vi "continuous_volumetric_scan.vi"() -> ()   [LabVIEW 2017]
uses:
  <vilib>/DAQmx/write.llb/DAQmx Write (Analog DBL 1Chan 1Samp).vi
  <vilib>/DAQmx/write.llb/DAQmx Write (Analog 1D DBL NChan 1Samp).vi
  <vilib>/DAQmx/write.llb/DAQmx Write (Analog 2D DBL NChan NSamp).vi
  <vilib>/DAQmx/create/channels.llb/DAQmx Create Channel (AO-Voltage-Basic).vi
  <vilib>/DAQmx/miscellaneous.llb/DAQmx Fill In Error Info.vi
  <vilib>/Utility/file.llb/Read Delimited Spreadsheet (DBL).vi
  <vilib>/measure/mascope.llb/Transition Measurements 1 chan.vi
  <vilib>/DAQmx/configure/timing.llb/DAQmx Timing (Sample Clock).vi
  <vilib>/DAQmx/configure/trigger.llb/DAQmx Start Trigger (Digital Edge).vi
  <vilib>/measure/NI_MAPro.lvlib
panel:
  out "Sampling rate":i32
  out "ETL3":waveform(dbl)(graph)
  out "mirror y":waveform(dbl)(graph)
  out "mirror x":waveform(dbl)(graph)
  out "561":waveform(dbl)(graph)
  out "488":waveform(dbl)(graph)
  out "camera":waveform(dbl)(graph)
  out "mirx transition duration":dbl
  out "transition duration":dbl
  out "etl3 timing array":dbl[](array[numeric])
  out "mirror y timing array":dbl[](array[numeric])
  out "mirror x timing array":dbl[](array[numeric])
  out "561 timing array":dbl[](array[numeric])
  out "488 timing array":dbl[](array[numeric])
  out "camera timing array":dbl[](array[numeric])
  out "etl raw":dbl[](array[numeric])
  out "miry raw":dbl[](array[numeric])
  out "mirx raw":dbl[](array[numeric])
  out "561 Intensity":dbl
  out "488 Intensity":dbl
  out "Off Time":dbl
  out "On Time":dbl
  out "Number of slices":dbl
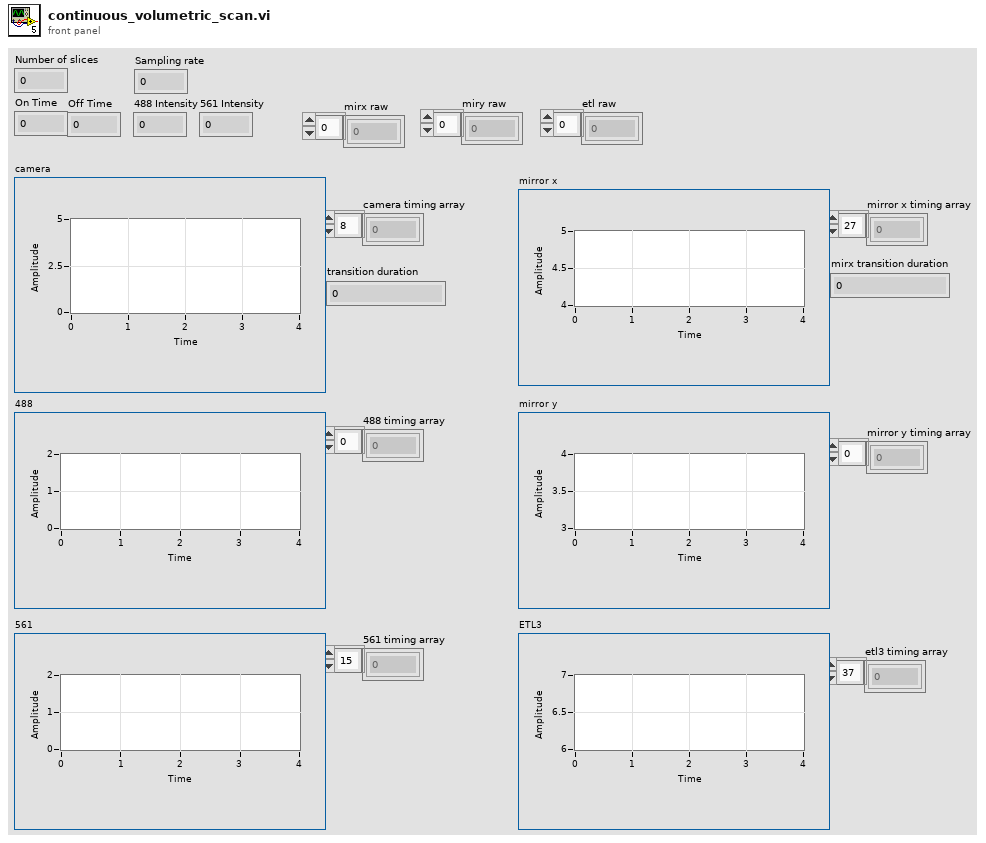
[diagram p1: front panel]
types:
  T1 = enum32{"Invalid", "Standard", "Closed", "Hidden", "Minimized", "Maximized"}
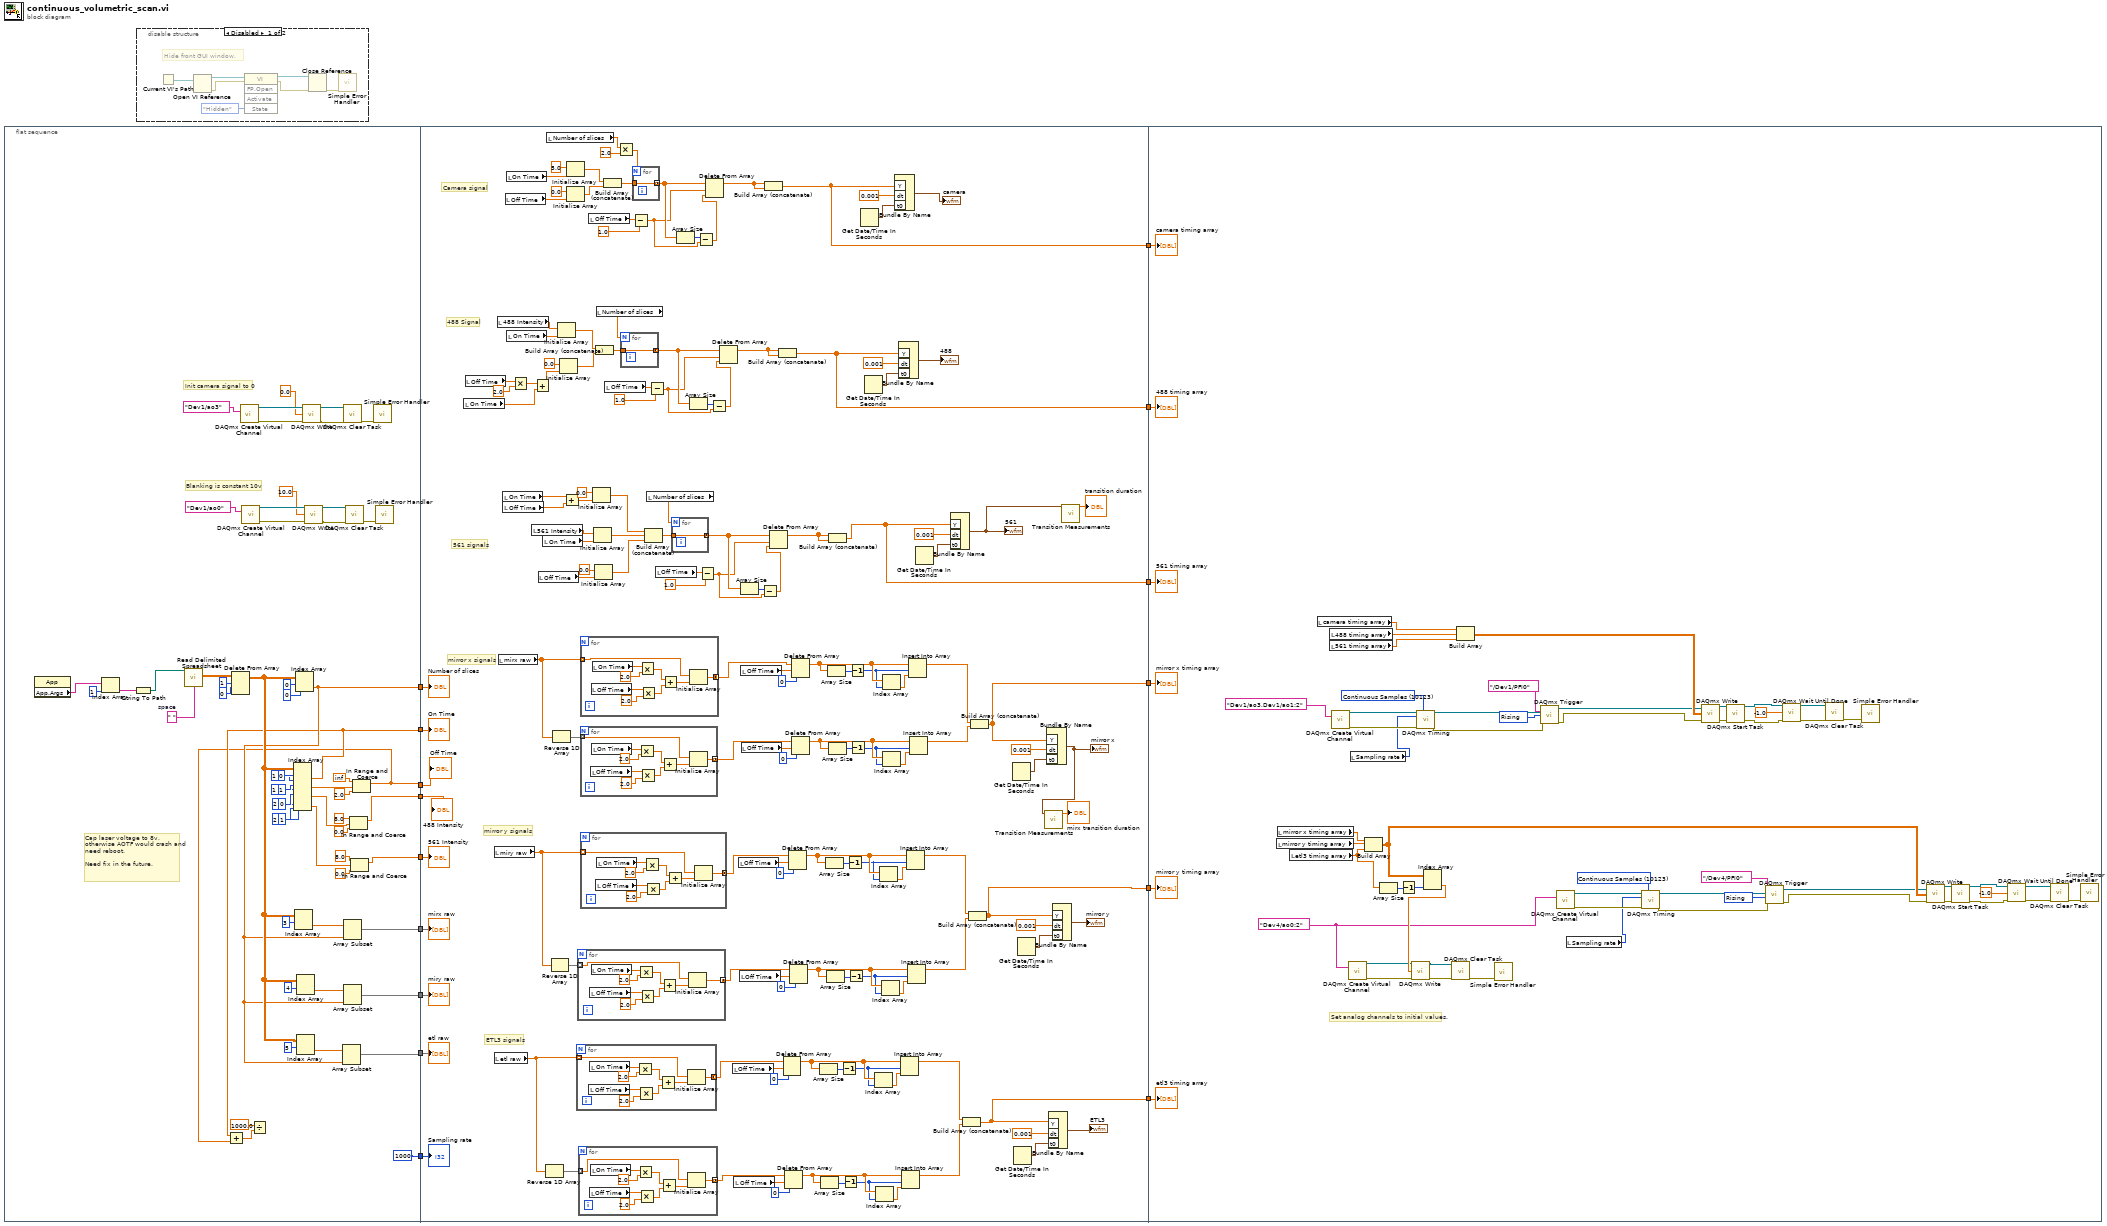
[diagram p0: block diagram]
diagram:
  n1 = flat-sequence {
    tunnel: [w50] -> w15
    tunnel: [w27] -> w14
    tunnel: [w26] -> w13
    tunnel: [w18] -> w12
    tunnel: [w16] -> w11
    tunnel: [w49] -> w10
    tunnel: [w48] -> w9
    tunnel: [w47] -> w8
    tunnel: [1000] -> w1
    tunnel: w15 -> [w97]
    tunnel: w14 -> [w96]
    tunnel: w13 -> [w95]
    tunnel: w12 -> [w94]
    tunnel: w11 -> [w93]
    tunnel: w10 -> [w92]
    tunnel: w9 -> [w91]
    tunnel: w8 -> [w90]
    tunnel: [w89] -> w7
    tunnel: [w88] -> w6
    tunnel: [w87] -> w5
    tunnel: [w86] -> w4
    tunnel: [w85] -> w3
    tunnel: [w84] -> w2
    tunnel: w1 -> [w75]
    tunnel: w7 -> [w288]
    tunnel: w6 -> [w287]
    tunnel: w5 -> [w286]
    tunnel: w4 -> [w285]
    tunnel: w3 -> [w284]
    tunnel: w2 -> [w283]
    frame #0 {
      w51 = " "  # space
      # "Cap laser voltage to 8v, otherwise AOTF would crash and need reboot. \n\nNeed fix in the future."
      # "Init camera signal to 0"
      # "Blanking is constant 10v"
      n2 = property class="App"() -> ("App.Args"=w30:string[])  [unwired: 2 in, 2 out]
      n3 = Index Array(array=w30, index=1) -> (element=w29:string)
      n4 = String To Path(string=w29) -> (path=w28:path)
      n5 = call-poly <vilib>:"Read Delimited Spreadsheet.vi"("file path (dialog if empty)"=w28, "delimiter (\\t)"=w51) -> ("all rows"=w69:dbl[][])  [unwired: 8 in, 5 out]
      n6 = Delete From Array(array=w69, length=1, index (row)=0) -> (array with subset deleted=w70:dbl[][])  [unwired: 1 in, 1 out]
      n7 = call-poly <vilib>:"DAQmx Create Virtual Channel.vi"("physical channels"=tag "Dev1/ao3") -> ("task out"=w35:refnum<k21>, "error out"=w36:errorcluster)  [unwired: 13 in]
      n8 = call-poly <vilib>:"DAQmx Create Virtual Channel.vi"("physical channels"=tag "Dev1/ao0") -> ("task out"=w43:refnum<k21>, "error out"=w44:errorcluster)  [unwired: 13 in]
      n9 = Index Array(array=w70, index (row) #1=1 ("index (row)"), index (col) #1=0 ("disabled index (col)"), index (row) #2=1 ("index (row)"), index (col) #2=1 ("disabled index (col)"), index (row) #3=2 ("index (row)"), index (col) #3=0 ("disabled index (col)"), index (row) #4=2 ("index (row)"), index (col) #4=1 ("disabled index (col)")) -> (element #1=w27:dbl, element #2=w74:dbl, element #3=w19:dbl, element #4=w17:dbl)
      n10 = Index Array(array=w70, index (row)=3) -> (element=w71:dbl[])  [unwired: 1 in]
      n11 = Index Array(array=w70, index (row)=0, index (col)=0 ("disabled index (col)")) -> (element=w50:dbl)
      n12 = Index Array(array=w70, index (row)=5) -> (element=w73:dbl[])  [unwired: 1 in]
      n13 = Index Array(array=w70, index (row)=4) -> (element=w72:dbl[])  [unwired: 1 in]
      n14 = call-poly <vilib>:"DAQmx Write.vi"("task/channels in"=w35, "data"=0.0, "error in"=w36) -> ("task out"=w37:refnum<k21>, "error out"=w38:errorcluster)  [unwired: 10 in, 1 out]
      n15 = call-poly <vilib>:"DAQmx Write.vi"("task/channels in"=w43, "data"=10.0, "error in"=w44) -> ("task out"=w45:refnum<k21>, "error out"=w46:errorcluster)  [unwired: 10 in, 1 out]
      n16 = Array Subset(array=w73, length=w50) -> (w47:dbl[])  [unwired: 1 in]
      n17 = call <vilib>:"DAQmx Clear Task.vi"("task in"=w37, "error in"=w38) -> ("error out"=w34:errorcluster)  [unwired: 13 in]
      n18 = Array Subset(array=w71, length=w50) -> (w49:dbl[])  [unwired: 1 in]
      n19 = Array Subset(array=w72, length=w50) -> (w48:dbl[])  [unwired: 1 in]
      n20 = call <vilib>:"DAQmx Clear Task.vi"("task in"=w45, "error in"=w46) -> ("error out"=w42:errorcluster)  [unwired: 13 in]
      n21 = In Range and Coerce(upper limit=8.0, x=w19, lower limit=0.0) -> (coerced(x)=w18:dbl)  [unwired: 1 out]
      n22 = In Range and Coerce(upper limit=8.0, x=w17, lower limit=0.0) -> (coerced(x)=w16:dbl)  [unwired: 1 out]
      n23 = In Range and Coerce(upper limit=inf, x=w74, lower limit=2.0) -> (coerced(x)=w26:dbl)  [unwired: 1 out]
      n24 = Add(x=w27, y=w26) -> (x+y=w24:dbl)
      n25 = Divide(x=1000.0, y=w24) -> ()  [unwired: 1 out]
      n26 = call <vilib>:"Simple Error Handler.vi"("error in (no error)"=w34) -> ()  [unwired: 4 in, 5 out]
      n27 = call <vilib>:"Simple Error Handler.vi"("error in (no error)"=w42) -> ()  [unwired: 4 in, 5 out]
    }
    frame #1 {
      # "ETL3 signals"
      # "mirror y signals"
      # "mirror x signals"
      # "561 signals"
      # "488 Signal"
      # "Camera signal"
      n28 = local read "On Time"() -> (w195:dbl)
      n29 = local read "Off Time"() -> (w198:dbl)
      n30 = local read "miry raw"() -> (w124:dbl[])
      n31 = local read "etl raw"() -> (w120:dbl[])
      n32 = local read "488 Intensity"() -> (w202:dbl)
      n33 = local read "mirx raw"() -> (w128:dbl[])
      n34 = local read "On Time"() -> (w169:dbl)
      n35 = local read "Off Time"() -> (w180:dbl)
      n36 = local read "Off Time"() -> (w217:dbl)
      n37 = local read "On Time"() -> (w218:dbl)
      n38 = local read "On Time"() -> (w201:dbl)
      n39 = Multiply(x=w198, y=2.0) -> (x*y=w196:dbl)
      n40 = local read "561 Intensity"() -> (w183:dbl)
      n41 = Add(x=w196, y=w195) -> (x+y=w194:dbl)
      n42 = local read "Off Time"() -> (w165:dbl)
      n43 = local read "On Time"() -> (w182:dbl)
      n44 = Reverse 1D Array(array=w120) -> (reversed array=w118:dbl[])
      n45 = local read "Number of slices"() -> (w210:dbl)
      n46 = Reverse 1D Array(array=w124) -> (reversed array=w122:dbl[])
      n47 = Reverse 1D Array(array=w128) -> (reversed array=w126:dbl[])
      n48 = Initialize Array(w202, w201) -> (w200:dbl[])
      n49 = Initialize Array(0.0 ("element"), w194) -> (w193:dbl[])
      n50 = Add(x=w169, y=w180) -> (x+y=w179:dbl)
      n51 = Initialize Array(5.0 ("element"), w218) -> (w215:dbl[])
      n52 = Initialize Array(0.0 ("element"), w217) -> (w214:dbl[])
      n53 = for {
        tunnel: w120 -> [w230] mode=indexing
        tunnel: [w229] -> w119 mode=concatenating
        n54 = local read "Off Time"() -> (w235:dbl)
        n55 = local read "On Time"() -> (w233:dbl)
        n56 = Multiply(x=w233, y=2.0) -> (x*y=w234:dbl)
        n57 = Multiply(x=w235, y=2.0) -> (x*y=w236:dbl)
        n58 = Add(x=w234, y=w236) -> (x+y=w237:dbl)
        n59 = Initialize Array(w230, w237) -> (w229:dbl[])
      }
      n60 = for {
        tunnel: w122 -> [w239] mode=indexing
        tunnel: [w238] -> w121 mode=concatenating
        n61 = local read "Off Time"() -> (w244:dbl)
        n62 = local read "On Time"() -> (w242:dbl)
        n63 = Multiply(x=w242, y=2.0) -> (x*y=w243:dbl)
        n64 = Multiply(x=w244, y=2.0) -> (x*y=w245:dbl)
        n65 = Add(x=w243, y=w245) -> (x+y=w246:dbl)
        n66 = Initialize Array(w239, w246) -> (w238:dbl[])
      }
      n67 = for {
        tunnel: w118 -> [w221] mode=indexing
        tunnel: [w220] -> w117 mode=concatenating
        n68 = local read "Off Time"() -> (w226:dbl)
        n69 = local read "On Time"() -> (w224:dbl)
        n70 = Multiply(x=w224, y=2.0) -> (x*y=w225:dbl)
        n71 = Multiply(x=w226, y=2.0) -> (x*y=w227:dbl)
        n72 = Add(x=w225, y=w227) -> (x+y=w228:dbl)
        n73 = Initialize Array(w221, w228) -> (w220:dbl[])
      }
      n74 = for {
        tunnel: w128 -> [w266] mode=indexing
        tunnel: [w265] -> w127 mode=concatenating
        n75 = local read "Off Time"() -> (w271:dbl)
        n76 = local read "On Time"() -> (w273:dbl)
        n77 = Multiply(x=w273, y=2.0) -> (x*y=w272:dbl)
        n78 = Multiply(x=w271, y=2.0) -> (x*y=w270:dbl)
        n79 = Add(x=w272, y=w270) -> (x+y=w269:dbl)
        n80 = Initialize Array(w266, w269) -> (w265:dbl[])
      }
      n81 = for {
        tunnel: w126 -> [w257] mode=indexing
        tunnel: [w256] -> w125 mode=concatenating
        n82 = local read "Off Time"() -> (w262:dbl)
        n83 = local read "On Time"() -> (w264:dbl)
        n84 = Multiply(x=w264, y=2.0) -> (x*y=w263:dbl)
        n85 = Multiply(x=w262, y=2.0) -> (x*y=w261:dbl)
        n86 = Add(x=w263, y=w261) -> (x+y=w260:dbl)
        n87 = Initialize Array(w257, w260) -> (w256:dbl[])
      }
      n88 = for {
        tunnel: w124 -> [w248] mode=indexing
        tunnel: [w247] -> w123 mode=concatenating
        n89 = local read "Off Time"() -> (w253:dbl)
        n90 = local read "On Time"() -> (w251:dbl)
        n91 = Multiply(x=w251, y=2.0) -> (x*y=w252:dbl)
        n92 = Multiply(x=w253, y=2.0) -> (x*y=w254:dbl)
        n93 = Add(x=w252, y=w254) -> (x+y=w255:dbl)
        n94 = Initialize Array(w248, w255) -> (w247:dbl[])
      }
      n95 = local read "Off Time"() -> (w209:dbl)
      n96 = Initialize Array(0.0 ("element"), w179) -> (w168:dbl[])
      n97 = Initialize Array(w183, w182) -> (w167:dbl[])
      n98 = Initialize Array(0.0 ("element"), w165) -> (w164:dbl[])
      n99 = Build Array (concatenate)(w200, w193) -> (w191:dbl[])
      n100 = local read "Number of slices"() -> (w192:dbl)
      n101 = Build Array (concatenate)(w215, w214) -> (w213:dbl[])
      n102 = local read "Off Time"() -> (w187:dbl)
      n103 = Multiply(x=w210, y=2.0) -> (x*y=w212:dbl)
      n104 = for {
        N: w192 -> [_]
        tunnel: w191 -> [w275]
        tunnel: [w275] -> w188 mode=concatenating
      }
      n105 = for {
        N: w212 -> [_]
        tunnel: w213 -> [w276]
        tunnel: [w276] -> w207 mode=concatenating
      }
      n106 = Subtract(x=w209, y=1.0) -> (x-y=w205:dbl)
      n107 = Build Array (concatenate)(w168, w167, w164) -> (w177:dbl[])
      n108 = local read "Number of slices"() -> (w178:dbl)
      n109 = Subtract(x=w187, y=1.0) -> (x-y=w185:dbl)
      n110 = local read "Off Time"() -> (w173:dbl)
      n111 = for {
        N: w178 -> [_]
        tunnel: w177 -> [w274]
        tunnel: [w274] -> w174 mode=concatenating
      }
      n112 = Array Size(array=w207) -> (size(s)=w206:i32)
      n113 = Array Size(array=w188) -> (size(s)=w190:i32)
      n114 = Subtract(x=w206, y=w205) -> (x-y=w204:dbl)
      n115 = Subtract(x=w173, y=1.0) -> (x-y=w171:dbl)
      n116 = Delete From Array(array=w207, length=w205, index=w204) -> (array with subset deleted=w203:dbl[])  [unwired: 1 out]
      n117 = Subtract(x=w190, y=w185) -> (x-y=w189:dbl)
      n118 = Delete From Array(array=w188, length=w185, index=w189) -> (array with subset deleted=w184:dbl[])  [unwired: 1 out]
      n119 = local read "Off Time"() -> (w139:dbl)
      n120 = local read "Off Time"() -> (w134:dbl)
      n121 = local read "Off Time"() -> (w151:dbl)
      n122 = local read "Off Time"() -> (w146:dbl)
      n123 = Array Size(array=w174) -> (size(s)=w176:i32)
      n124 = local read "Off Time"() -> (w163:dbl)
      n125 = local read "Off Time"() -> (w158:dbl)
      n126 = Subtract(x=w176, y=w171) -> (x-y=w175:dbl)
      n127 = Build Array (concatenate)(w203, w203) -> (w89:dbl[])
      n128 = Delete From Array(array=w174, length=w171, index=w175) -> (array with subset deleted=w170:dbl[])  [unwired: 1 out]
      n129 = Build Array (concatenate)(w184, w184) -> (w88:dbl[])
      n130 = Delete From Array(array=w119, length=w139, index=0) -> (array with subset deleted=w136:dbl[])  [unwired: 1 out]
      n131 = Delete From Array(array=w117, length=w134, index=0) -> (array with subset deleted=w131:dbl[])  [unwired: 1 out]
      n132 = Delete From Array(array=w123, length=w151, index=0) -> (array with subset deleted=w148:dbl[])  [unwired: 1 out]
      n133 = Delete From Array(array=w121, length=w146, index=0) -> (array with subset deleted=w143:dbl[])  [unwired: 1 out]
      n134 = Delete From Array(array=w127, length=w163, index=0) -> (array with subset deleted=w160:dbl[])  [unwired: 1 out]
      n135 = Delete From Array(array=w125, length=w158, index=0) -> (array with subset deleted=w155:dbl[])  [unwired: 1 out]
      n136 = Array Size(array=w136) -> (size(s)=w138:i32)
      n137 = Array Size(array=w131) -> (size(s)=w133:i32)
      n138 = Array Size(array=w148) -> (size(s)=w150:i32)
      n139 = Array Size(array=w143) -> (size(s)=w145:i32)
      n140 = Array Size(array=w160) -> (size(s)=w162:i32)
      n141 = Array Size(array=w155) -> (size(s)=w157:i32)
      n142 = Build Array (concatenate)(w170, w170) -> (w87:dbl[])
      n143 = Decrement(x=w138) -> (x-1=w135:i32)
      n144 = Decrement(x=w133) -> (x-1=w130:i32)
      n145 = Decrement(x=w150) -> (x-1=w147:i32)
      n146 = Decrement(x=w145) -> (x-1=w142:i32)
      n147 = Decrement(x=w162) -> (x-1=w159:i32)
      n148 = Decrement(x=w157) -> (x-1=w154:i32)
      n149 = Get Date/Time In Seconds() -> (seconds since 1Jan1904=w111:timestamp)
      n150 = Get Date/Time In Seconds() -> (seconds since 1Jan1904=w109:timestamp)
      n151 = Index Array(array=w136, index=w135) -> (element=w137:dbl)
      n152 = Index Array(array=w131, index=w130) -> (element=w132:dbl)
      n153 = Index Array(array=w148, index=w147) -> (element=w149:dbl)
      n154 = Index Array(array=w143, index=w142) -> (element=w144:dbl)
      n155 = Index Array(array=w160, index=w159) -> (element=w161:dbl)
      n156 = Index Array(array=w155, index=w154) -> (element=w156:dbl)
      n157 = Bundle By Name("Y"=w89, "dt"=0.001, "t0"=w111) -> (→"camera":waveform(dbl))  [unwired: 1 in]
      n158 = Bundle By Name("Y"=w88, "dt"=0.001, "t0"=w109) -> (→"488":waveform(dbl))  [unwired: 1 in]
      n159 = Insert Into Array(array=w136, index=w135, new element=w137) -> (w129:dbl[])
      n160 = Insert Into Array(array=w131, index=w130, new element=w132) -> (w104:dbl[])
      n161 = Insert Into Array(array=w148, index=w147, new element=w149) -> (w141:dbl[])
      n162 = Insert Into Array(array=w143, index=w142, new element=w144) -> (w140:dbl[])
      n163 = Insert Into Array(array=w160, index=w159, new element=w161) -> (w153:dbl[])
      n164 = Insert Into Array(array=w155, index=w154, new element=w156) -> (w152:dbl[])
      n165 = Get Date/Time In Seconds() -> (seconds since 1Jan1904=w113:timestamp)
      n166 = Bundle By Name("Y"=w87, "dt"=0.001, "t0"=w113) -> (w79:waveform(dbl))  [unwired: 1 in]
      "561" <- w79
      n167 = Build Array (concatenate)(w129, w104) -> (w84:dbl[])
      n168 = Build Array (concatenate)(w141, w140) -> (w85:dbl[])
      n169 = Build Array (concatenate)(w153, w152) -> (w86:dbl[])
      n170 = Get Date/Time In Seconds() -> (seconds since 1Jan1904=w115:timestamp)
      n171 = Get Date/Time In Seconds() -> (seconds since 1Jan1904=w105:timestamp)
      n172 = Get Date/Time In Seconds() -> (seconds since 1Jan1904=w107:timestamp)
      n173 = Bundle By Name("Y"=w86, "dt"=0.001, "t0"=w115) -> (w78:waveform(dbl))  [unwired: 1 in]
      "mirror x" <- w78
      n174 = call-poly <vilib>:"Transition Measurements.vi"("signal in"=w78) -> ("transition duration"=→"mirx transition duration":dbl)  [unwired: 5 in, 5 out]
      n175 = Bundle By Name("Y"=w84, "dt"=0.001, "t0"=w105) -> (→"ETL3":waveform(dbl))  [unwired: 1 in]
      n176 = Bundle By Name("Y"=w85, "dt"=0.001, "t0"=w107) -> (→"mirror y":waveform(dbl))  [unwired: 1 in]
      n177 = call-poly <vilib>:"Transition Measurements.vi"("signal in"=w79) -> ("transition duration"=→"transition duration":dbl)  [unwired: 5 in, 5 out]
      "Number of slices" <- w97
      "On Time" <- w96
      "Off Time" <- w95
      "488 Intensity" <- w94
      "561 Intensity" <- w93
      "mirx raw" <- w92
      "miry raw" <- w91
      "etl raw" <- w90
      "Sampling rate" <- w75
    }
    frame #2 {
      w297 = 10280 items=["Rising"=10280, "Falling"=10171] ("edge")
      w294 = 10123 items=["Finite Samples"=10178, "Continuous Samples"=10123, "Hardware Timed Single Point"=12522] ("sample mode")
      w296 = tag "Dev4/ao0:2" ("physical channels")
      w292 = 10280 items=["Rising"=10280, "Falling"=10171] ("edge")
      w289 = 10123 items=["Finite Samples"=10178, "Continuous Samples"=10123, "Hardware Timed Single Point"=12522] ("sample mode")
      # "Set analog channels to initial values."
      n178 = local read "mirror y timing array"() -> (w317:dbl[])
      n179 = local read "mirror x timing array"() -> (w318:dbl[])
      n180 = local read "etl3 timing array"() -> (w335:dbl[])
      n181 = local read "camera timing array"() -> (w315:dbl[])
      n182 = local read "488 timing array"() -> (w314:dbl[])
      n183 = local read "561 timing array"() -> (w319:dbl[])
      n184 = call-poly <vilib>:"DAQmx Create Virtual Channel.vi"("physical channels"=tag "Dev1/ao3,Dev1/ao1:2") -> ("task out"=w306:refnum<k21>, "error out"=w307:errorcluster)  [unwired: 13 in]
      n185 = call-poly <vilib>:"DAQmx Create Virtual Channel.vi"("physical channels"=w296) -> ("task out"=w310:refnum<k21>, "error out"=w311:errorcluster)  [unwired: 13 in]
      n186 = local read "Sampling rate"() -> (w282:i32)
      n187 = Build Array(w318, w317, w335) -> (w334:dbl[][])
      n188 = Array Size(array=w335) -> (size(s)=w320:i32)
      n189 = Decrement(x=w320) -> (x-1=w321:i32)
      n190 = call-poly <vilib>:"DAQmx Timing.vi"("task/channels in"=w306, "sample mode"=w289, "rate"=w282, "error in"=w307) -> ("task out"=w308:refnum<k21>, "error out"=w309:errorcluster)  [unwired: 10 in]
      n191 = Index Array(array=w334, index (col)=w321) -> (element=w322:dbl[])  [unwired: 1 in]
      n192 = call-poly <vilib>:"DAQmx Write.vi"("task/channels in"=w310, "data"=w322, "error in"=w311) -> ("task out"=w312:refnum<k21>, "error out"=w313:errorcluster)  [unwired: 10 in, 1 out]
      n193 = call <vilib>:"DAQmx Clear Task.vi"("task in"=w312, "error in"=w313) -> ("error out"=w336:errorcluster)  [unwired: 13 in]
      n194 = Build Array(w315, w314, w319) -> (w316:dbl[][])
      n195 = call <vilib>:"Simple Error Handler.vi"("error in (no error)"=w336) -> ()  [unwired: 4 in, 5 out]
      n196 = call-poly <vilib>:"DAQmx Trigger.vi"("task/channels in"=w308, "source"=tag "/Dev1/PFI0", "edge"=w292, "error in"=w309) -> ("task out"=w280:refnum<k21>, "error out"=w279:errorcluster)  [unwired: 10 in]
      n197 = call-poly <vilib>:"DAQmx Create Virtual Channel.vi"("physical channels"=w296) -> ("task out"=w330:refnum<k21>, "error out"=w331:errorcluster)  [unwired: 13 in]
      n198 = local read "Sampling rate"() -> (w281:i32)
      n199 = call-poly <vilib>:"DAQmx Timing.vi"("task/channels in"=w330, "sample mode"=w294, "rate"=w281, "error in"=w331) -> ("task out"=w332:refnum<k21>, "error out"=w333:errorcluster)  [unwired: 10 in]
      n200 = call-poly <vilib>:"DAQmx Write.vi"("task/channels in"=w280, "data"=w316, "error in"=w279) -> ("task out"=w304:refnum<k21>, "error out"=w305:errorcluster)  [unwired: 10 in, 1 out]
      n201 = call <vilib>:"DAQmx Start Task.vi"("task/channels in"=w304, "error in"=w305) -> ("task out"=w303:refnum<k21>, "error out"=w302:errorcluster)  [unwired: 12 in]
      n202 = call-poly <vilib>:"DAQmx Trigger.vi"("task/channels in"=w332, "source"=tag "/Dev4/PFI0", "edge"=w297, "error in"=w333) -> ("task out"=w278:refnum<k21>, "error out"=w277:errorcluster)  [unwired: 10 in]
      n203 = call <vilib>:"DAQmx Wait Until Done.vi"("task/channels in"=w303, "timeout (sec)"=-1.0, "error in"=w302) -> ("task out"=w300:refnum<k21>, "error out"=w301:errorcluster)  [unwired: 11 in]
      n204 = call <vilib>:"DAQmx Clear Task.vi"("task in"=w300, "error in"=w301) -> ("error out"=w299:errorcluster)  [unwired: 13 in]
      n205 = call <vilib>:"Simple Error Handler.vi"("error in (no error)"=w299) -> ()  [unwired: 4 in, 5 out]
      n206 = call-poly <vilib>:"DAQmx Write.vi"("task/channels in"=w278, "data"=w334, "error in"=w277) -> ("task out"=w328:refnum<k21>, "error out"=w329:errorcluster)  [unwired: 10 in, 1 out]
      n207 = call <vilib>:"DAQmx Start Task.vi"("task/channels in"=w328, "error in"=w329) -> ("task out"=w327:refnum<k21>, "error out"=w326:errorcluster)  [unwired: 12 in]
      n208 = call <vilib>:"DAQmx Wait Until Done.vi"("task/channels in"=w327, "timeout (sec)"=-1.0, "error in"=w326) -> ("task out"=w324:refnum<k21>, "error out"=w325:errorcluster)  [unwired: 11 in]
      n209 = call <vilib>:"DAQmx Clear Task.vi"("task in"=w324, "error in"=w325) -> ("error out"=w323:errorcluster)  [unwired: 13 in]
      n210 = call <vilib>:"Simple Error Handler.vi"("error in (no error)"=w323) -> ()  [unwired: 4 in, 5 out]
      "camera timing array" <- w288
      "488 timing array" <- w287
      "561 timing array" <- w286
      "mirror x timing array" <- w285
      "mirror y timing array" <- w284
      "etl3 timing array" <- w283
    }
  }
  n211 = disable-structure shown="Disabled" {
    frame Disabled {
      # "Hide front GUI window."
      n212 = Current VI's Path() -> (path=w343:path)
      n213 = Open VI Reference(vi path=w343) -> (vi reference=w341:refnum<vi>, error out=w340:errorcluster)  [unwired: 5 in]
      n214 = invoke class="VI" method="FP.Open"(reference=w341, error in=w340, "State"=T1."Hidden") -> (reference out=w339:refnum<vi>, error out=w338:errorcluster)  [unwired: 2 in, 3 out]
      n215 = Close Reference(reference=w339, error in (no error)=w338) -> (error out=w342:errorcluster)
      n216 = call <vilib>:"Simple Error Handler.vi"("error in (no error)"=w342) -> ()  [unwired: 4 in, 5 out]
    }
    frame Enabled {
    }
  }
